vi "get_number_of_blocks.vi"(8 "error in (no error)":errorcluster, 11 "GenericWriteSignals in":refnum<class "GenericSignalWriter.lvclass">) -> (0 "error out":errorcluster, 2 "number of blocks":i32, 3 "GenericWriteSignals out":refnum<class "GenericSignalWriter.lvclass">)   [LabVIEW 2010, in "GenericSignalWriter.lvclass"]
uses:
  GenericSignalWriter.lvclass
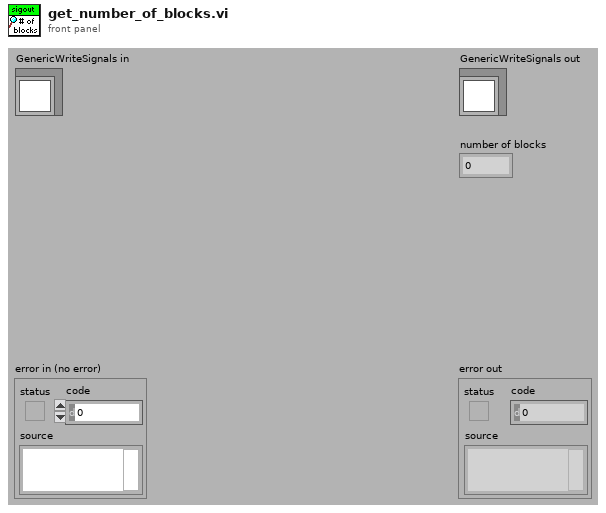
[diagram p1: front panel]
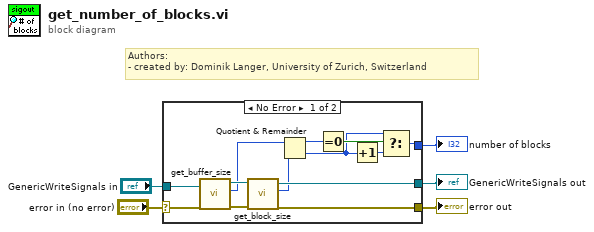
[diagram p0: block diagram]
diagram:
  # "Authors: \n- created by: Dominik Langer, University of Zurich, Switzerland"
  n1 = case shown="No Error" "error in (no error)" {
    selector: "error in (no error)" -> [w14 w20]
    tunnel: [w13 w20] -> w4
    tunnel: [w15 w19] -> w2
    tunnel: "GenericWriteSignals in" -> [w18 w19]
    tunnel: [w6 _] -> w1
    frame No Error {
      n2 = call-dynamic "get_buffer_size.vi"("error in (no error)"=w14, "GenericWriteSignals.lvclass in"=w18) -> ("error out"=w17:errorcluster, "buffer size (samples)"=w12:i32, "GenericWriteSignals.lvclass out"=w16:refnum<class "GenericSignalWriter.lvclass">)  [unwired: 7 out]
      n3 = call "get_block_size.vi"("error in (no error)"=w17, "GenericWriteSignals.lvclass in"=w16) -> ("error out"=w13:errorcluster, "block size"=w11:i32, "GenericWriteSignals.lvclass out"=w15:refnum<class "GenericSignalWriter.lvclass">)  [unwired: 7 out]
      n4 = Quotient & Remainder(x=w12, y=w11) -> (x-y*floor(x/y)=w10:i32, floor(x/y)=w8:i32)
      n5 = Equal To 0?(x=w10) -> (x = 0?=w9:bool)
      n6 = Increment(x=w8) -> (x+1=w7:i32)
      n7 = Select(t=w8, s=w9, f=w7) -> (s? t:f=w6:i32)
    }
    frame Error {
    }
  }
  "error out" <- w4
  "GenericWriteSignals out" <- w2
  "number of blocks" <- w1
